vi "Untitled 6.vi"() -> ()   [LabVIEW 2010]
uses:
  <vilib>/NXT/Block Support/NXT_InputPort.ctl
  <vilib>/NXT/Subs/MotorOutput.ctl
  <vilib>/NXT/Dual Mode Library/Sensors/Light_On.vi
  <vilib>/NXT/Dual Mode Library/Motors/MotorBrake.vi
  <vilib>/NXT/Dual Mode Library/Motors/MotorOn.vi
panel:
  in  "오른쪽모터":T1=3 caption="Output Port" items=["Port A", "Port B", "Port C", "All Ports"]
  in  "왼쪽모터":T1=3 caption="Output Port" items=["Port A", "Port B", "Port C", "All Ports"]
  in  "stop 2":bool
  in  "stop":bool
  in  "?":i32=75
  in  "Output Port (All Ports) 2":T1=3 items=["Port A", "Port B", "Port C", "All Ports"]
  in  "오른쪽 빛센서":T2=2 caption="Port (Port 3)" items=["Port 1", "Port 2", "Port 3", "Port 4"]
  in  "Output Port (All Ports)":T1=3 items=["Port A", "Port B", "Port C", "All Ports"]
  in  "?":i32=75
  in  "왼쪽 빛센서":T2=2 caption="Port (Port 3)" items=["Port 1", "Port 2", "Port 3", "Port 4"]
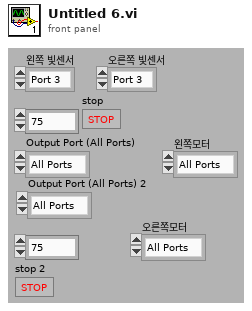
[diagram p1: front panel]
types:
  T1 = typedef "MotorOutput.ctl" = u8
  T2 = typedef "NXT_InputPort.ctl" = u8
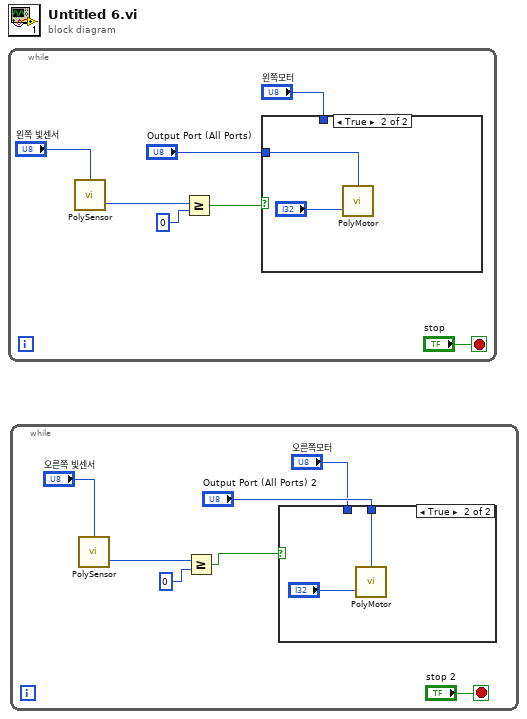
[diagram p0: block diagram]
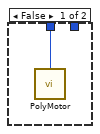
[diagram p2: hidden frame]
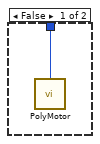
[diagram p3: hidden frame]
diagram:
  n1 = while {
    stop <- "stop" stop-if-true
    n2 = call-poly <vilib>:"PolySensor.vi"("Port (Port 3)"="왼쪽 빛센서") -> ("Scaled Value"=w6:i16)  [unwired: 2 in, 1 out]
    n3 = Greater Or Equal?(x=w6, y=i16 0) -> (x >= y?=w4:bool)
    n4 = case shown="True" w4 {
      tunnel: "Output Port (All Ports)" -> [_ w9]
      tunnel: "왼쪽모터" -> [w8 _]
      frame False {
        n5 = call-poly <vilib>:"PolyMotor.vi"("Port (All Ports)"=w8) -> ()  [unwired: 3 in, 1 out]
      }
      frame True {
        n6 = call-poly <vilib>:"PolyMotor.vi"("Power (75)"="?", "Output Port (All Ports)"=w9) -> ()  [unwired: 2 in, 1 out]
      }
    }
  }
  n7 = while {
    stop <- "stop 2" stop-if-true
    n8 = call-poly <vilib>:"PolySensor.vi"("Port (Port 3)"="오른쪽 빛센서") -> ("Scaled Value"=w16:i16)  [unwired: 2 in, 1 out]
    n9 = Greater Or Equal?(x=w16, y=i16 0) -> (x >= y?=w14:bool)
    n10 = case shown="True" w14 {
      tunnel: "Output Port (All Ports) 2" -> [_ w20]
      tunnel: "오른쪽모터" -> [w18 _]
      frame False {
        n11 = call-poly <vilib>:"PolyMotor.vi"("Port (All Ports)"=w18) -> ()  [unwired: 3 in, 1 out]
      }
      frame True {
        n12 = call-poly <vilib>:"PolyMotor.vi"("Power (75)"="?", "Output Port (All Ports)"=w20) -> ()  [unwired: 2 in, 1 out]
      }
    }
  }
